vi "AddErrorToMap.vi"(2 "Error reported":errorcluster, 5 "Error In":errorcluster) -> (19 "Error Out":errorcluster)   [LabVIEW 2018, in "Error handler.lvclass"]
uses:
  Error handler.lvclass
panel:
  # "Missing object. The object \"Map\" does not exist in the previous version."
  # "Missing object. The object \"Map\" does not exist in the previous version."
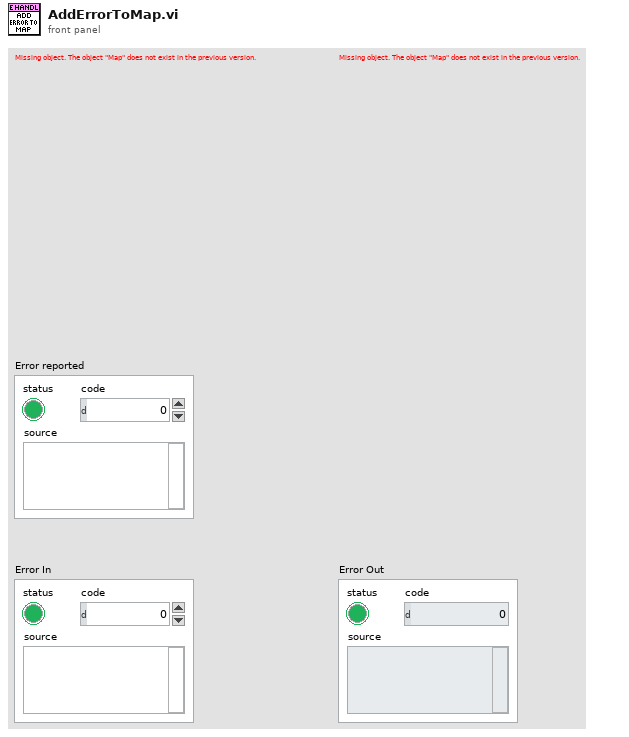
[diagram p1: front panel]
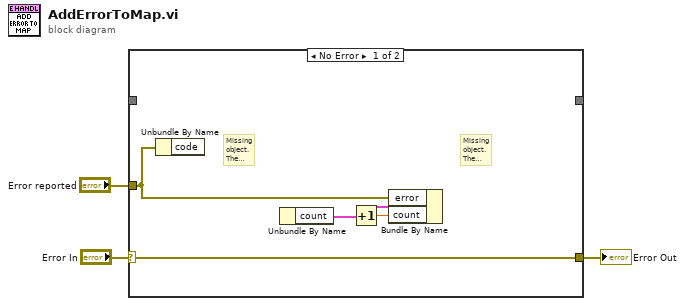
[diagram p0: block diagram]
diagram:
  n1 = case shown="No Error" "Error In" {
    selector: "Error In" -> [w14 w16]
    tunnel: [w14 w16] -> w4
    tunnel: [w13 w15] -> w3
    tunnel: [w12 w15] -> w2
    tunnel: "Error reported" -> [w9 _]
    frame No Error {
      # "Missing object. The object \"Look In Map\" does not exist in the previous version."
      # "Missing object. The object \"Insert Into Map\" does not exist in the previous version."
      n2 = Unbundle By Name(w9) -> ("code"=w11:i32)
      n3 = Unbundle By Name(w8) -> ("count"=w7)
      n4 = Increment(x=w7) -> (x+1=w6:dbl)
      n5 = Bundle By Name("error"=w9, "count"=w6) -> (w10:cluster{}, w8:cluster{})
    }
    frame Error {
    }
  }
  "Error Out" <- w4
